vi "get_freq.vi"(8 "approx freq":dbl, 9 "ch to get":i32, 11 "wavemeter cluster":cluster{"Cur Ch":i32, "Frequency":dbl}) -> (3 "Frequency":dbl)   [LabVIEW 2012]
doc: "Returns the frequency for the specified chanel given a cluster of ch and freq. Must be within 0.1 THz of approx freq to return. Otherwise returns the last reading.\nIs reentrant."
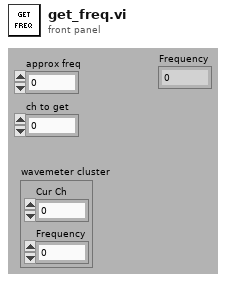
[diagram p1: front panel]
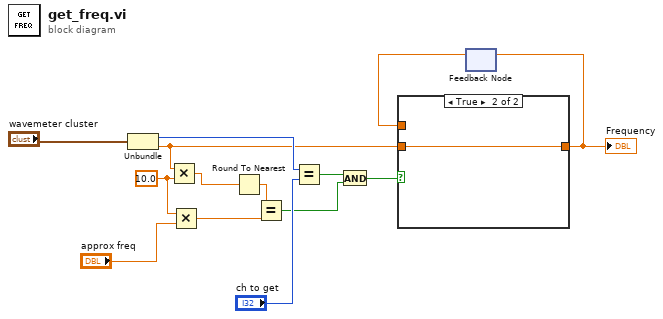
[diagram p0: block diagram]
diagram:
  w1 = 10.0 ("y")
  n1 = Unbundle("wavemeter cluster") -> ("Cur Ch"=w13:i32, "Frequency"=w5:dbl)
  n2 = Multiply(x=w5, y=w1) -> (x*y=w4:dbl)
  n3 = Multiply(x=w1, y="approx freq") -> (x*y=w2:dbl)
  n4 = Round To Nearest(number=w4) -> (nearest integer value=w10:dbl)
  n5 = Equal?(x=w10, y=w2) -> (x = y?=w9:bool)
  n6 = Equal?(x=w13, y="ch to get") -> (x = y?=w11:bool)
  n7 = And(x=w11, y=w9) -> (x .and. y?=w8:bool)
  n8 = feedback #1() -> (w6:dbl)  [unwired: 1 in]
  n9 = case shown="True" w8 {
    tunnel: w5 -> [_ w16]
    tunnel: [w15 w16] -> w7
    tunnel: w6 -> [w15 _]
    frame False {
    }
    frame True {
    }
  }
  "Frequency" <- w7
  n10 = feedback-in #1(w7) -> ()
